vi "BRig_RT__Case_Exp__storeData__endExp__v5__p3__v2__wait.vi"(7 "input_True":bool=TRUE, 9 "input_dataAnalog":u16[][](array[numeric]), 12 "input_count":i32) -> (8 "output_True":bool)   [LabVIEW 2014]
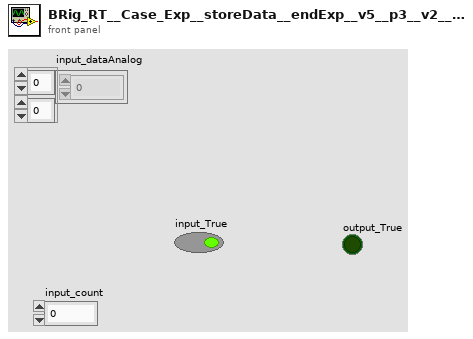
[diagram p1: front panel]
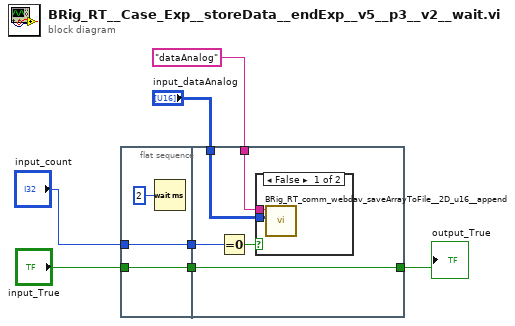
[diagram p0: block diagram]
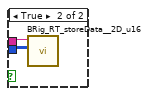
[diagram p2: hidden frame]
diagram:
  n1 = flat-sequence {
    tunnel: [w10] -> w5
    tunnel: "input_True" -> [w10]
    tunnel: "input_count" -> [w9]
    tunnel: [w9] -> w1
    tunnel: "input_dataAnalog" -> [w13]
    tunnel: "dataAnalog" ("input_filename") -> [w15]
    tunnel: w5 -> [w14]
    tunnel: [w14] -> w4
    tunnel: w1 -> [w11]
    frame #0 {
      n2 = Wait (ms)(milliseconds to wait=u32 2) -> ()  [unwired: 1 out]
    }
    frame #1 {
      n3 = Equal To 0?(x=w11) -> (x = 0?=w12:bool)
      n4 = case shown="False" w12 {
        tunnel: w15 -> [w17 w19]
        tunnel: w13 -> [w16 w18]
        frame False {
          n5 = call "BRig_RT_comm_webdav_saveArrayToFile__2D_u16__append.vi"("Array"=w16, "input_filename"=w17) -> ()  [unwired: 10 in]
        }
        frame True {
          n6 = call "BRig_RT_storeData__2D_u16.vi"("Array"=w18, "input_filename"=w19) -> ()  [unwired: 10 in]
        }
      }
    }
  }
  "output_True" <- w4
